vi "Guitar with leds from 2 part live feed.vi"() -> ()   [LabVIEW 2009]
uses:
  <vilib>/vision/Image Controls.llb/IMAQ Image.ctl
  <vilib>/Instr/_visa.llb/VISA Configure Serial Port (Instr).vi
  <vilib>/userDefined/High Color/IMAQdx.ctl
  <vilib>/Analysis/3filter.llb/Filter Passband Type.ctl
  <vilib>/Analysis/3filter.llb/Butterworth Filter (DBL).vi
  <vilib>/vision/driver/NI_Vision_Acquisition_Software.lvlib
  <vilib>/Analysis/NI_AALBase.lvlib
  <vilib>/vision/NI_Vision_Development_Module.lvlib
panel:
  out "cluster":T1
  in  "baud rate (9600)":u32=9600
  in  "VISA resource name":refnum<visa-resource-name>
  out "number":u32
  out "decimal integer string":string
  in  "stop 3":bool
  out "Image":T2(plugin-control)
  out "Image Dst Out":T2
  in  "frame rate":dbl=29.97
  in  "sampling":dbl=1.0 format="%0.2f"
  in  "high":dbl=60.0 format="%0.2f"
  out "Waveform RED":dbl[](graph)
  in  "low":dbl=0.12500000000000006 format="%0.4f"
  out "LED RED":bool
  out "Waveform BLUE":dbl[](graph)
  out "LED BLUE":bool
  in  "sampling 2":dbl=1.0 format="%0.2f"
  in  "high 2":dbl=60.0 format="%0.2f"
  in  "low  2":dbl=0.12500000000000006 format="%0.4f"
  out "Red Line":T3={"Global Rectangle"=[168, 264, 180, 378], "Contours"=[{"ID"=enum."External", "Type"=2, "Coordinates"=[168, 377, 179, 264]}]} {"Contours"."Type" items=["No Selection", "Point", "Line", "Rectangle", "Oval", "Polygon", "Freehand Region", "Annulus", "Unused2", "Unused3", "Broken Line", "Freehand Line", "Rotated Rectangle"]}
  out "Blue Line":T3={"Global Rectangle"=[243, 262, 261, 384], "Contours"=[{"ID"=enum."External", "Type"=2, "Coordinates"=[260, 383, 243, 262]}]} {"Contours"."Type" items=["No Selection", "Point", "Line", "Rectangle", "Oval", "Polygon", "Freehand Region", "Annulus", "Unused2", "Unused3", "Broken Line", "Freehand Line", "Rotated Rectangle"]}
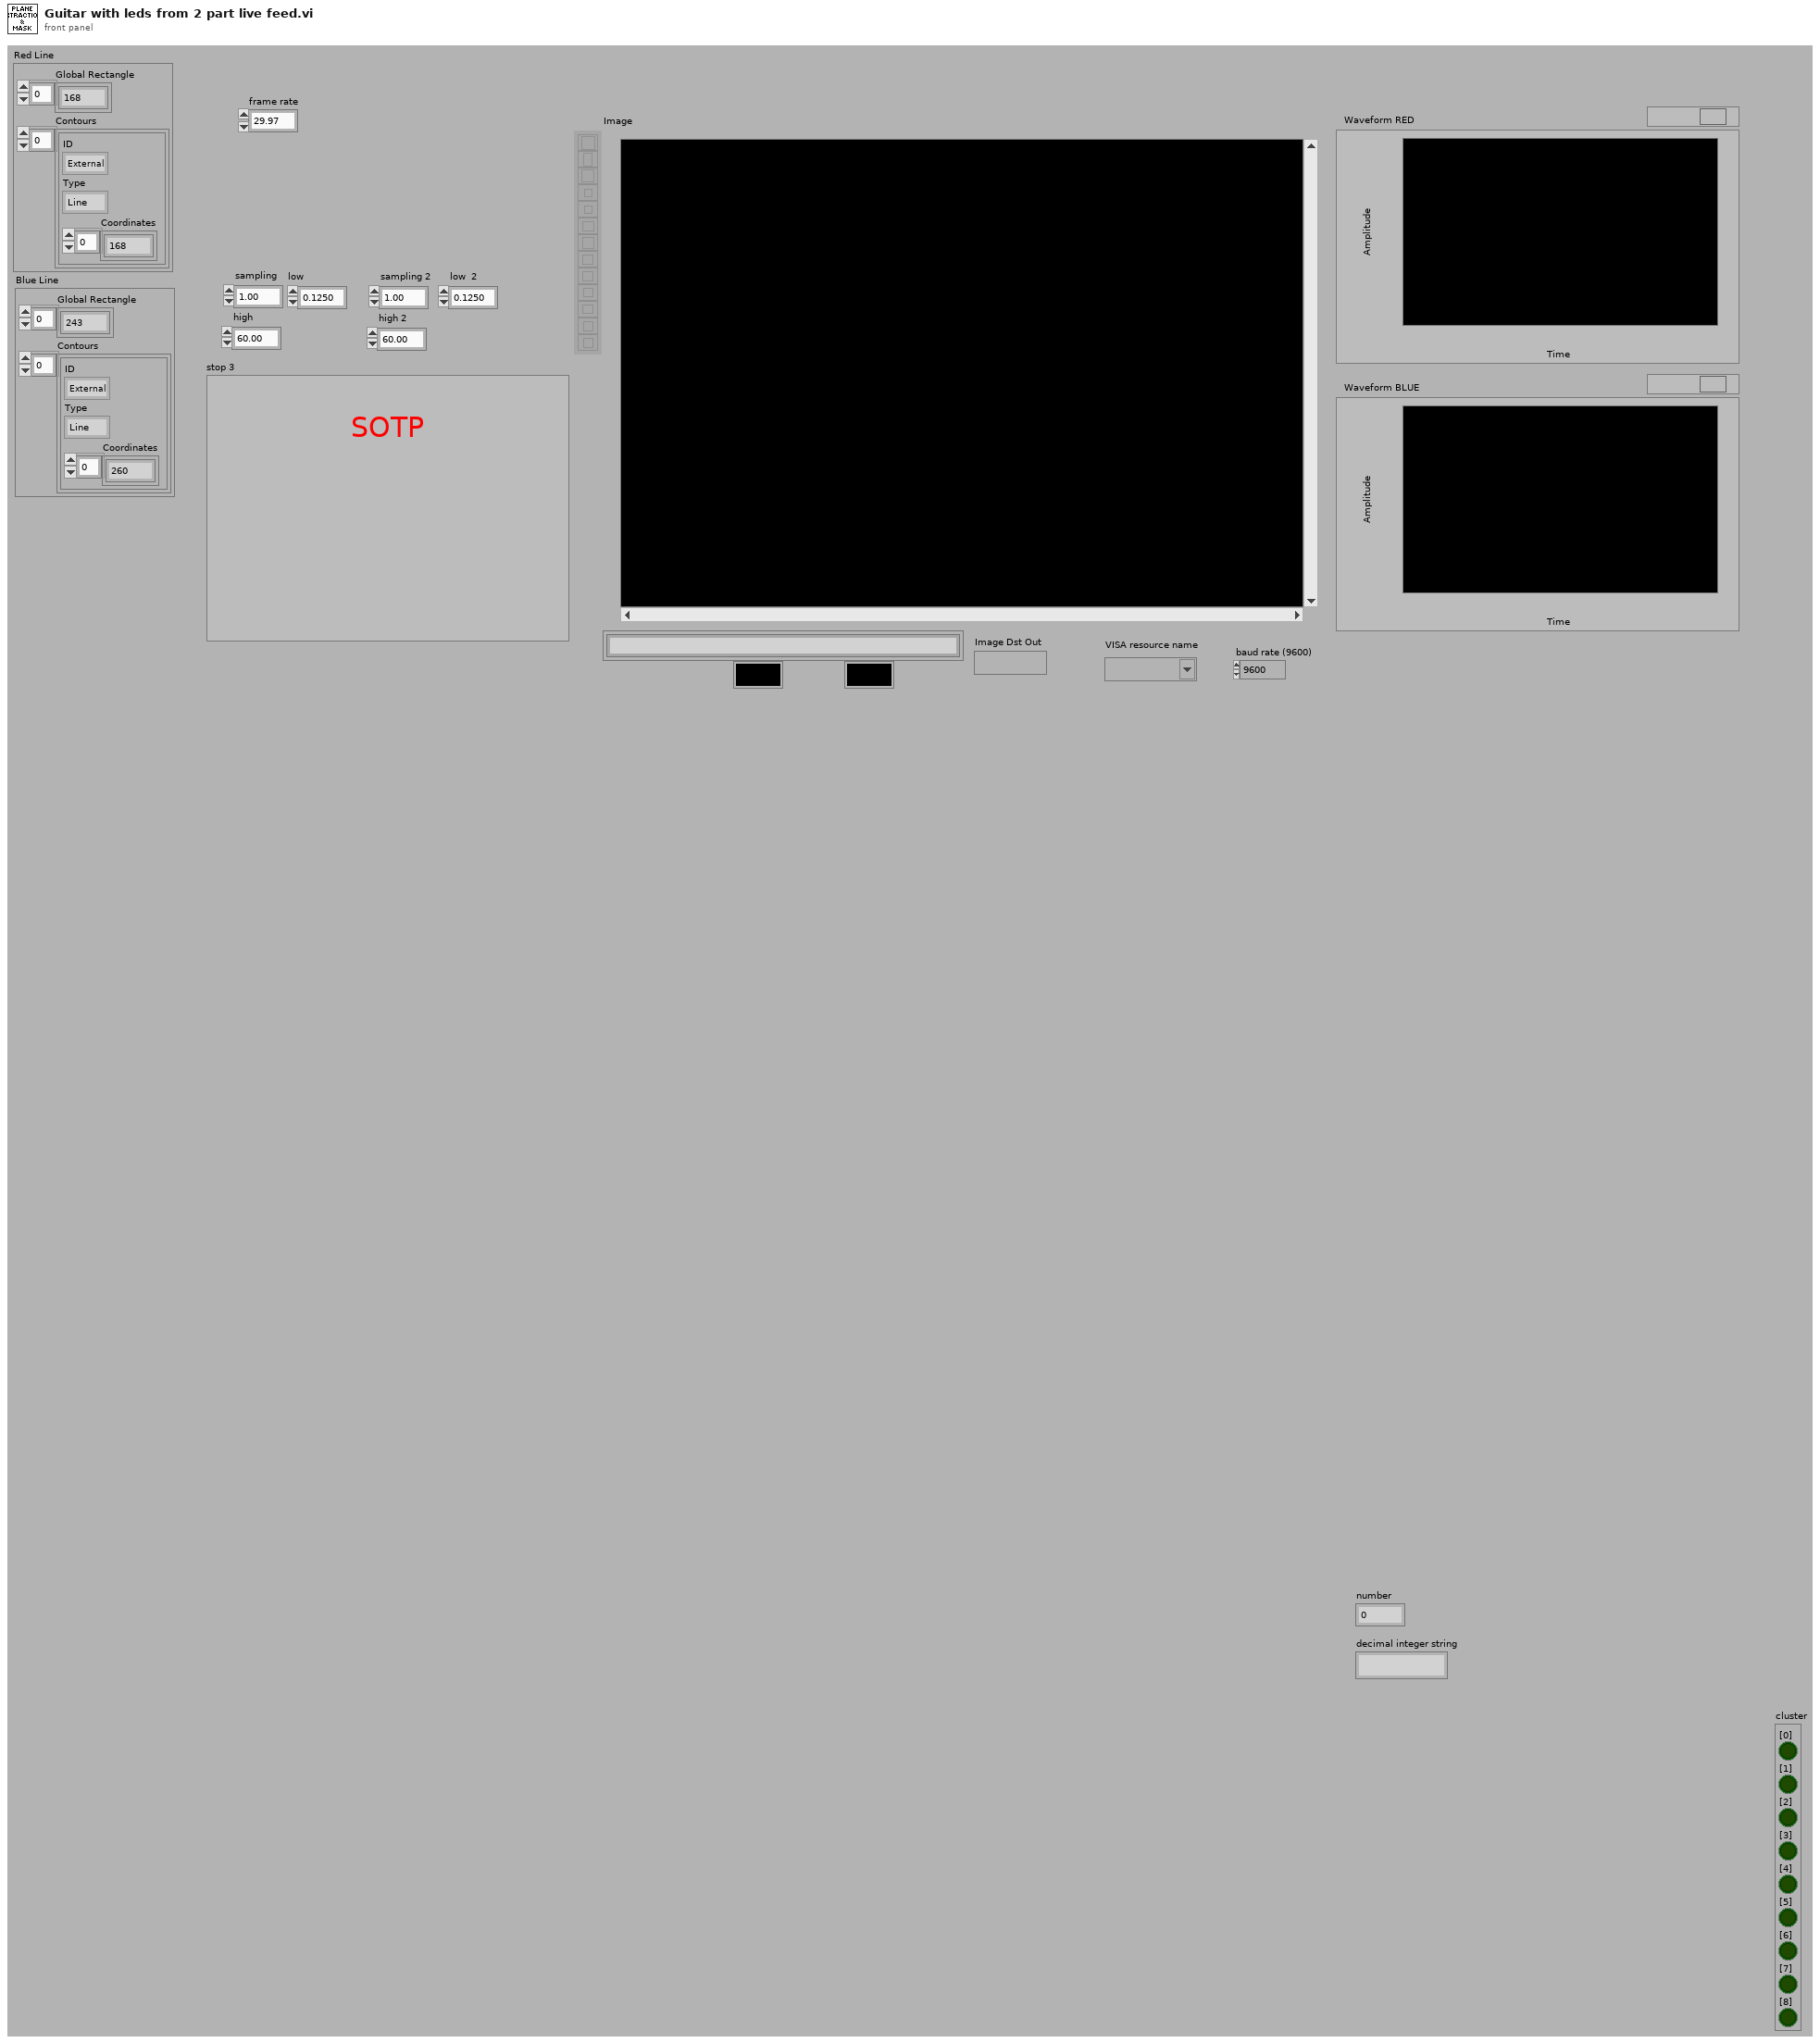
[diagram p1: front panel]
types:
  T1 = cluster{"[0]":bool, "[1]":bool, "[2]":bool, "[3]":bool, "[4]":bool, "[5]":bool, "[6]":bool, "[7]":bool, "[8]":bool}
  T2 = typedef "IMAQ Image.ctl" = refnum<image>
  T3 = cluster{"Global Rectangle":i32[], "Contours":cluster{"ID":enum32{"External", "Internal"}, "Type":u32, "Coordinates":i32[]}[]}
  T4 = typedef "IMAQdx.ctl" = refnum<k21>
  T5 = typedef "NI_AALBase.lvlib/Filter Passband Type.ctl" = enum32{"Lowpass", "Highpass", "Bandpass", "Bandstop"}
  T6 = cluster{"Left":i32, "Top":i32, "Right":i32, "Bottom":i32}
  T7 = typedef "Image Type" = u32
  T8 = cluster{"ID":enum32{"External", "Internal"}, "Type":u32, "Coordinates":i32[]}[]
  T9 = cluster{"ID":enum32{"External", "Internal"}, "Type":u32, "Coordinates":i32[]}
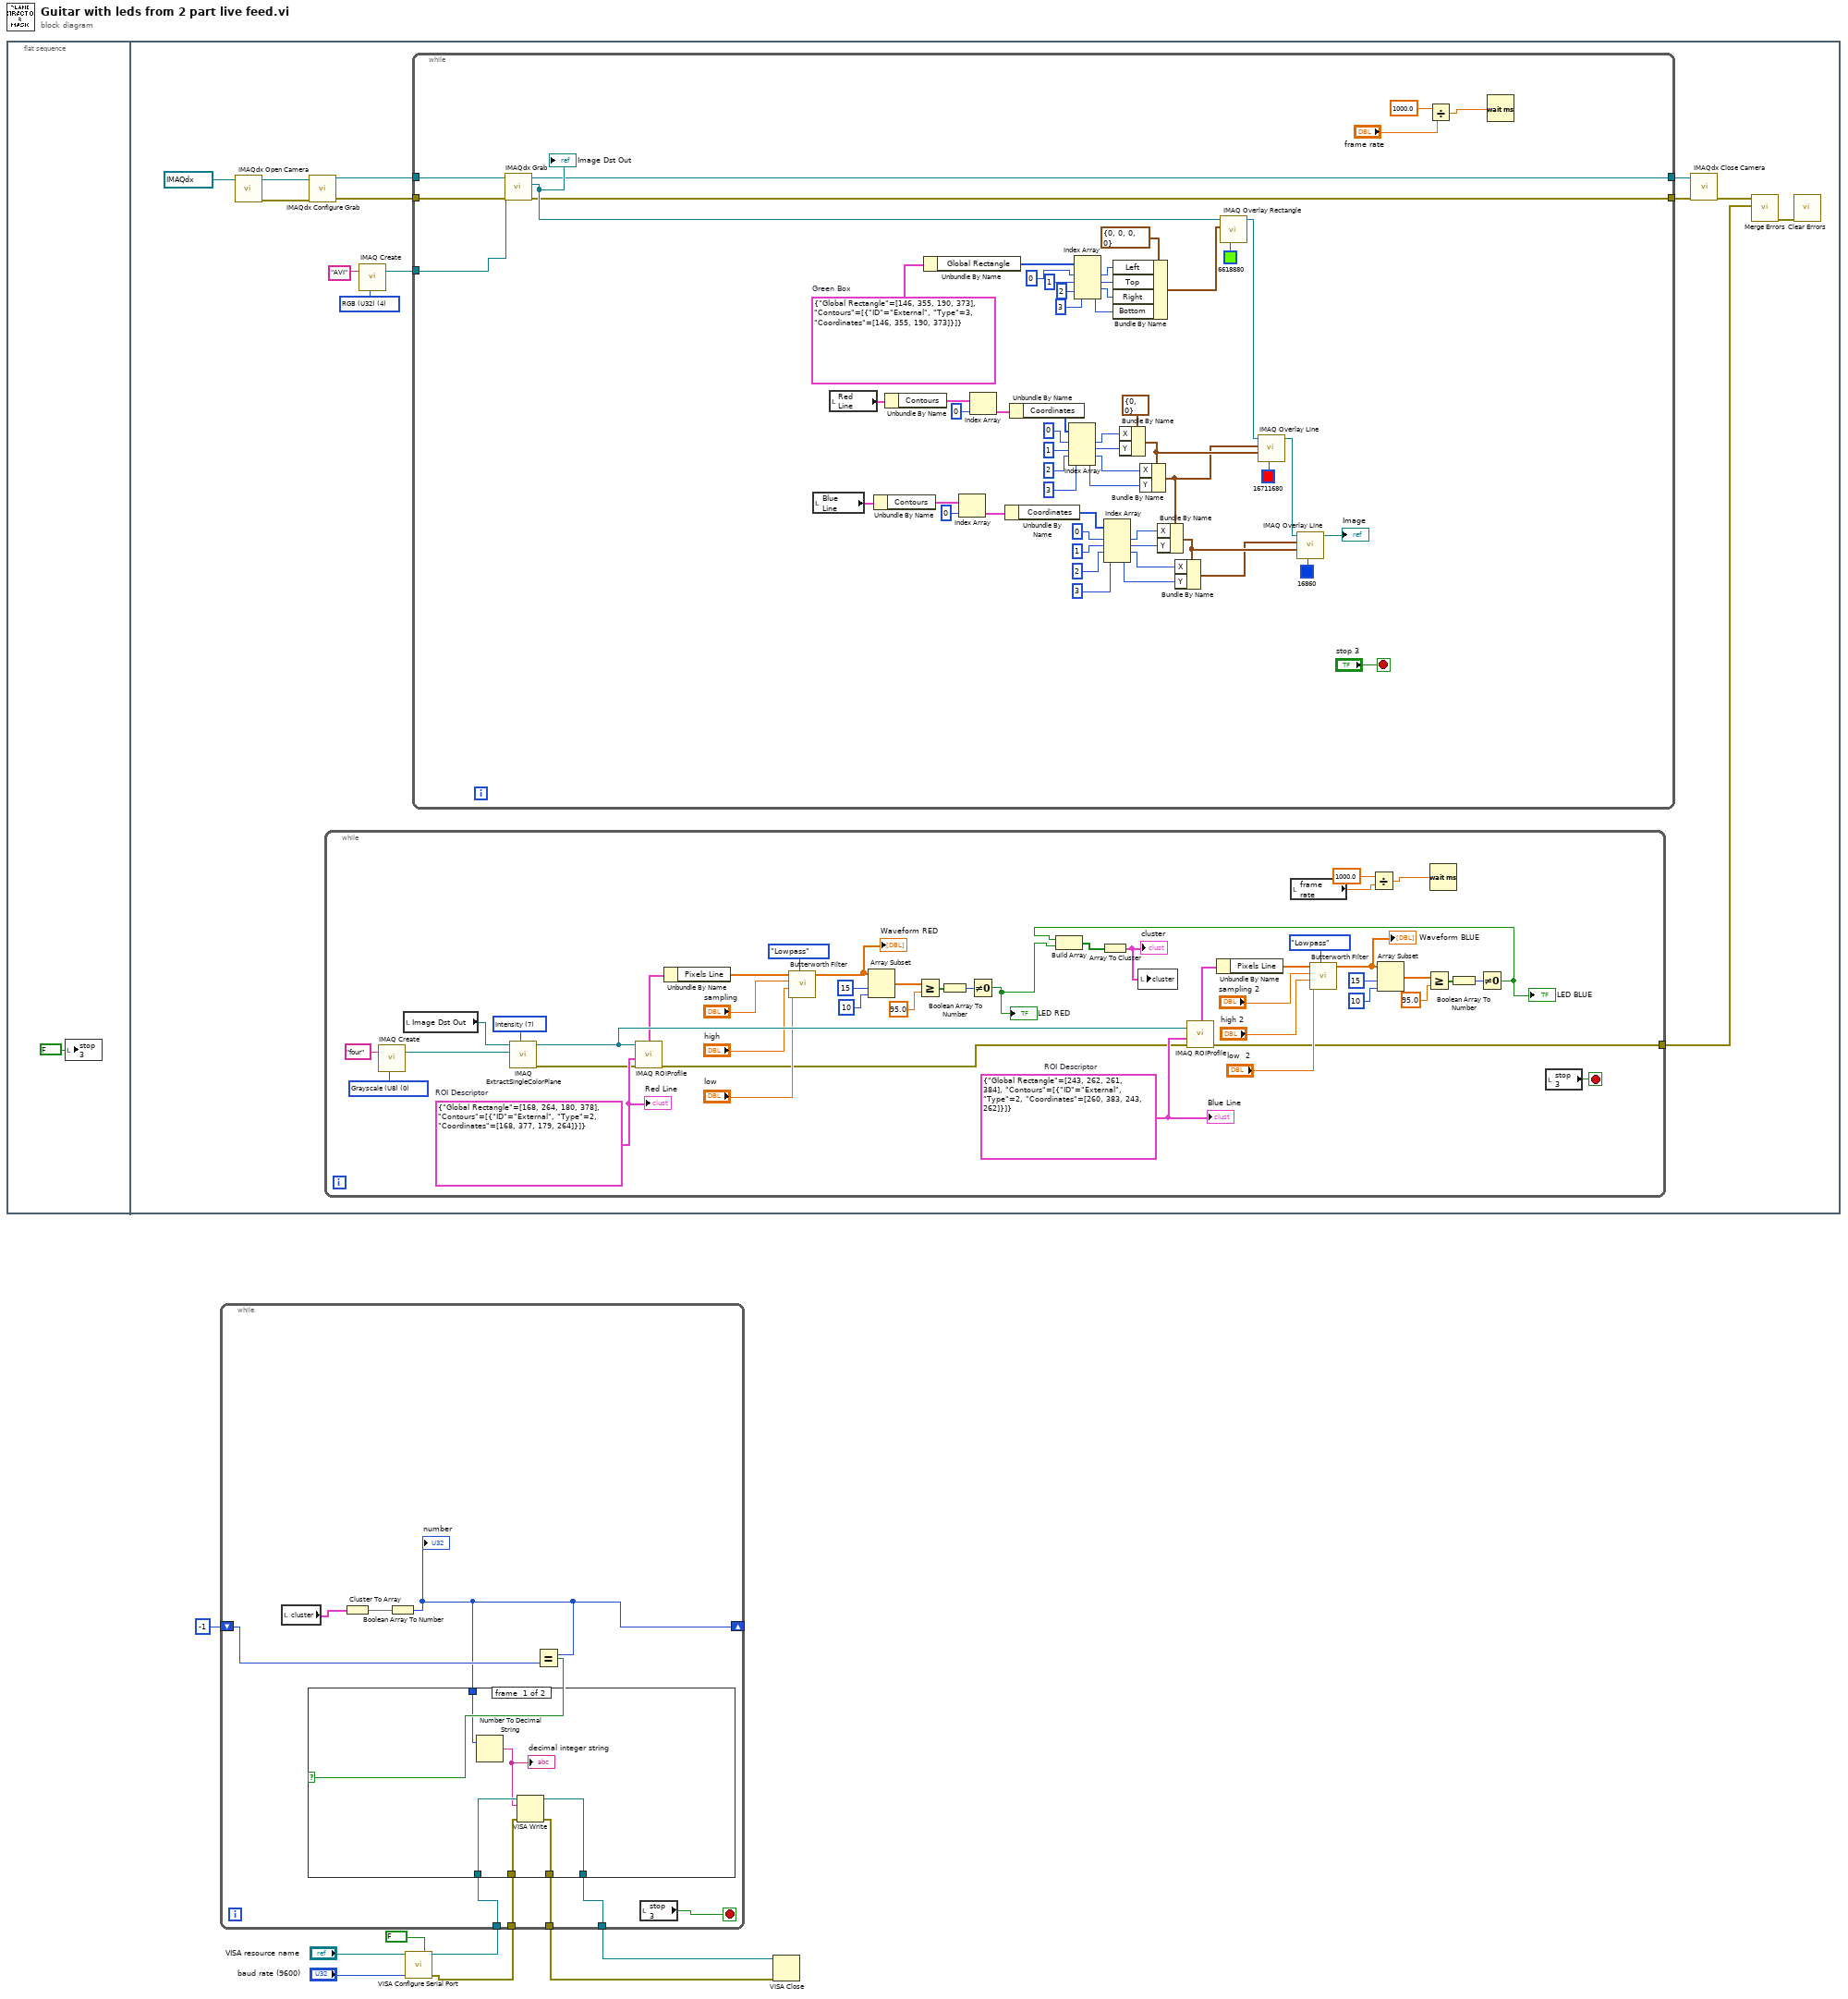
[diagram p0: block diagram]
diagram:
  n1 = flat-sequence {
    frame #0 {
      n2 = local write "stop 3"(FALSE ("stop")) -> ()
    }
    frame #1 {
      w12 = T7 4 items=["Grayscale (U8)", "Grayscale (I16)", "Grayscale (SGL)", "Complex (CSG)", "RGB (U32)", "HSL (U32)", "RGB (U64)", "Grayscale (U16)"] ("Image Type")
      n3 = call <vilib>:"IMAQdx Open Camera.vi"("Session In"=T4 "cam1") -> ("error out"=w18:errorcluster, "Session Out"=w19:T4)  [unwired: 9 in]
      n4 = call <vilib>:"IMAQdx Configure Grab.vi"("error in"=w18, "Session In"=w19) -> ("error out"=w16:errorcluster, "Session Out"=w17:T4)  [unwired: 8 in]
      n5 = while {
        tunnel: [w33] -> w22
        stop <- w65 stop-if-true
        w32 = T7 0 items=["Grayscale (U8)", "Grayscale (I16)", "Grayscale (SGL)", "Complex (CSG)", "RGB (U32)", "HSL (U32)", "RGB (U64)", "Grayscale (U16)"] ("Image Type")
        w63 = T3 {"Global Rectangle"=[243, 262, 261, 384], "Contours"=[{"ID"=enum."External", "Type"=2, "Coordinates"=[260, 383, 243, 262]}]}  # ROI Descriptor
        w64 = T3 {"Global Rectangle"=[168, 264, 180, 378], "Contours"=[{"ID"=enum."External", "Type"=2, "Coordinates"=[168, 377, 179, 264]}]}  # ROI Descriptor
        w67 = 7 items=["Red", "Green", "Blue", "Hue", "Saturation", "Luminance", "Value", "Intensity"] ("Color Plane")
        n6 = call "IMAQ Create"("Image Name"="four", "Image Type"=w32) -> ("New Image"=w30:T2)  [unwired: 3 in, 1 out]
        n7 = local read "Image Dst Out"() -> (w35:T2)
        n8 = call "IMAQ ExtractSingleColorPlane"("Color Plane"=w67, "Image Dst"=w30, "Image Src"=w35) -> ("error out"=w34:errorcluster, "Image Dst Out"=w66:T2)  [unwired: 1 in, 6 out]
        n9 = call "IMAQ ROIProfile"("error in (no error)"=w34, "ROI Descriptor"=w64, "Image"=w66) -> ("error out"=w36:errorcluster, "ROI Graph"=w61:cluster{"x0":sgl, "dx":sgl, "Pixels Line":sgl[]})  [unwired: 4 out]
        n10 = Unbundle By Name(w61) -> ("Pixels Line"=w60:sgl[])
        n11 = call-poly <vilib>:"Butterworth Filter.vi"("filter type"=Filter_Passband_Type."Lowpass", "low cutoff freq: fl"="low", "high cutoff freq: fh"="high", "sampling freq: fs"="sampling", "X"=w60) -> ("Filtered X"=w56:dbl[])  [unwired: 3 in, 1 out]
        "Waveform RED" <- w56
        n12 = Array Subset(array=w56, index=15, length=10) -> (w53:dbl[])
        n13 = Greater Or Equal?(x=w53, y=95.0) -> (x >= y?=w51:bool[])
        n14 = Boolean Array To Number(Boolean array=w51) -> (number=w50:u32)
        n15 = Not Equal To 0?(x=w50) -> (x != 0?=w26:bool)
        "LED RED" <- w26
        n16 = call "IMAQ ROIProfile"("error in (no error)"=w36, "ROI Descriptor"=w63, "Image"=w66) -> ("error out"=w33:errorcluster, "ROI Graph"=w39:cluster{"x0":sgl, "dx":sgl, "Pixels Line":sgl[]})  [unwired: 4 out]
        n17 = Unbundle By Name(w39) -> ("Pixels Line"=w42:sgl[])
        n18 = local read "frame rate"() -> (w27:dbl)
        n19 = call-poly <vilib>:"Butterworth Filter.vi"("filter type"=Filter_Passband_Type."Lowpass", "low cutoff freq: fl"="low  2", "high cutoff freq: fh"="high 2", "sampling freq: fs"="sampling 2", "X"=w42) -> ("Filtered X"=w38:dbl[])  [unwired: 3 in, 1 out]
        "Waveform BLUE" <- w38
        n20 = Divide(x=1000.0, y=w27) -> (x/y=w28:dbl)
        n21 = Array Subset(array=w38, index=15, length=10) -> (w47:dbl[])
        n22 = Greater Or Equal?(x=w47, y=95.0) -> (x >= y?=w45:bool[])
        n23 = Wait (ms)(milliseconds to wait=w28) -> ()  [unwired: 1 out]
        n24 = Boolean Array To Number(Boolean array=w45) -> (number=w44:u32)
        n25 = Not Equal To 0?(x=w44) -> (x != 0?=w25:bool)
        "LED BLUE" <- w25
        n26 = Build Array(w25, w26) -> (w24:bool[])
        n27 = Array To Cluster(array=w24) -> (cluster=w23:T1)
        "cluster" <- w23
        n28 = local write "cluster"(w23) -> ()
        n29 = local read "stop 3"() -> (w65:bool)
        "Red Line" <- w64
        "Blue Line" <- w63
      }
      n30 = call "IMAQ Create"("Image Name"="AVI", "Image Type"=w12) -> ("New Image"=w10:T2)  [unwired: 3 in, 1 out]
      n31 = while {
        tunnel: [w75] -> w13
        tunnel: [w74] -> w14
        tunnel: w17 -> [w73]
        tunnel: w16 -> [w72]
        tunnel: w10 -> [w68]
        stop <- "stop 3" stop-if-true
        w125 = T3 {"Global Rectangle"=[146, 355, 190, 373], "Contours"=[{"ID"=enum."External", "Type"=3, "Coordinates"=[146, 355, 190, 373]}]}  # Green Box
        n32 = call <vilib>:"IMAQdx Grab.vi"("error in"=w72, "Image In"=w68, "Session In"=w73) -> ("error out"=w74:errorcluster, "Image Out"=w76:T2, "Session Out"=w75:T4)  [unwired: 5 in, 1 out]
        "Image Dst Out" <- w76
        n33 = local read "Blue Line"() -> (w78:T3)
        n34 = local read "Red Line"() -> (w77:T3)
        n35 = Unbundle By Name(w78) -> ("Contours"=w92:T8)
        n36 = Unbundle By Name(w77) -> ("Contours"=w107:T8)
        n37 = Unbundle By Name(w125) -> ("Global Rectangle"=w121:i32[])
        n38 = Index Array(array=w92, index=0) -> (element=w91:T9)
        n39 = Index Array(array=w107, index=0) -> (element=w109:T9)
        n40 = Unbundle By Name(w91) -> ("Coordinates"=w90:i32[])
        n41 = Unbundle By Name(w109) -> ("Coordinates"=w110:i32[])
        n42 = Index Array(array=w110, index #1=0 ("index"), index #2=1 ("index"), index #3=2 ("index"), index #4=3 ("index")) -> (element #1=w102:i32, element #2=w103:i32, element #3=w104:i32, element #4=w105:i32)
        n43 = Index Array(array=w121, index #1=0 ("index"), index #2=1 ("index"), index #3=2 ("index"), index #4=3 ("index")) -> (element #1=w120:i32, element #2=w119:i32, element #3=w118:i32, element #4=w117:i32)
        n44 = Index Array(array=w90, index #1=0 ("index"), index #2=1 ("index"), index #3=2 ("index"), index #4=3 ("index")) -> (element #1=w89:i32, element #2=w95:i32, element #3=w94:i32, element #4=w93:i32)
        n45 = Bundle By Name(cluster=T6 {"Left"=0, "Top"=0, "Right"=0, "Bottom"=0} ("Rectangle"), "Left"=w120, "Top"=w119, "Right"=w118, "Bottom"=w117) -> (w123:T6)
        n46 = Bundle By Name(cluster=cluster{"X":i32, "Y":i32} {"X"=0, "Y"=0} ("End Point"), "X"=w102, "Y"=w103) -> (w111:cluster{"X":i32, "Y":i32})
        n47 = Bundle By Name(cluster=w111, "X"=w104, "Y"=w105) -> (w81:cluster{"X":i32, "Y":i32})
        n48 = Bundle By Name(cluster=w81, "X"=w89, "Y"=w95) -> (w96:cluster{"X":i32, "Y":i32})
        n49 = Bundle By Name(cluster=w96, "X"=w94, "Y"=w93) -> (w87:cluster{"X":i32, "Y":i32})
        n50 = call "IMAQ Overlay Rectangle"("Color"=u32 6618880, "Rectangle"=w123, "Image"=w76) -> ("Image Out"=w97:T2)  [unwired: 7 in, 1 out]
        n51 = call "IMAQ Overlay Line"("Color"=u32 16711680, "End Point"=w111, "Start Point"=w81, "Image"=w97) -> ("Image Out"=w86:T2)  [unwired: 6 in, 1 out]
        n52 = call "IMAQ Overlay Line"("Color"=u32 16860, "End Point"=w96, "Start Point"=w87, "Image"=w86) -> ("Image Out"=→"Image":T2)  [unwired: 6 in, 1 out]
        n53 = Divide(x=1000.0, y="frame rate") -> (x/y=w71:dbl)
        n54 = Wait (ms)(milliseconds to wait=w71) -> ()  [unwired: 1 out]
      }
      n55 = call <vilib>:"IMAQdx Close Camera.vi"("error in"=w14, "Session In"=w13) -> ("error out"=w15:errorcluster)  [unwired: 9 in]
      n56 = call <vilib>:"Merge Errors.vi"("error in 2 (no error)"=w22, "error in 1 (no error)"=w15) -> ("error out"=w21:errorcluster)  [unwired: 5 in]
      n57 = call <vilib>:"Clear Errors.vi"("error in (no error)"=w21) -> ()  [unwired: 6 in, 1 out]
    }
  }
  n58 = call-poly "VISA Configure Serial Port"("VISA resource name"="VISA resource name", "Enable Termination\nChar (T)"=FALSE ("Enable Termination\nChar (T)"), "baud rate (9600)"="baud rate (9600)") -> ("VISA resource name out"=w7:refnum<visa-resource-name>, "error out"=w2:errorcluster)  [unwired: 11 in]
  n59 = while {
    shift-right: [w130] -> _
    shift-left: -1 -> [w136]
    tunnel: w7 -> [w134]
    tunnel: [w133] -> w6
    tunnel: w2 -> [w132]
    tunnel: [w131] -> w1
    stop <- w127 stop-if-true
    n60 = local read "cluster"() -> (w129:T1)
    n61 = Cluster To Array(cluster=w129) -> (array=w128:bool[])
    n62 = Boolean Array To Number(Boolean array=w128) -> (number=w130:u32)
    "number" <- w130
    n63 = Equal?(x=w130, y=w136) -> (x = y?=w135:bool)
    n64 = case shown="False" w135 {
      tunnel: w134 -> [w142 w144]
      tunnel: [w141 w144] -> w133
      tunnel: w130 -> [w139 _]
      tunnel: w132 -> [w138 w143]
      tunnel: [w137 w143] -> w131
      frame #0 {
        n65 = Number To Decimal String(number=w139) -> (decimal integer string=w140:string)  [unwired: 1 in]
        "decimal integer string" <- w140
        n66 = VISA Write(VISA resource name=w142, write buffer=w140, error in (no error)=w138) -> (VISA resource name out=w141:refnum<visa-resource-name>, error out=w137:errorcluster)  [unwired: 1 out]
      }
      frame #1 {
      }
    }
    n67 = local read "stop 3"() -> (w127:bool)
  }
  n68 = VISA Close(VISA resource name=w6, error in (no error)=w1) -> ()  [unwired: 1 out]
